vi "1.vi"() -> ()   [LabVIEW 2020]
uses:
  <vilib>/Native 3D Graph/xcontrol/3DPC_SurfacePlot.xctl
  <vilib>/imath/engines/lvmath2/RunTimeEngine/NodeEndStatement/NIMS_NodeEndStatement_Output.vi
  <instcachedir>/0/NIMS_NodeEndStatement_Output_53EC0D466D134D7ABD903AC30B43404B.lvgen/NIMS_NodeEndStatement_Output_53EC0D466D134D7ABD903AC30B43404B_005.vi
  <vilib>/imath/engines/lvmath2/RunTimeEngine/ErrorHandling/NIMS_Finalize Error.vi
  <instcachedir>/0/NIMS_NodeEndStatement_Output_53EC0D466D134D7ABD903AC30B43404B.lvgen/NIMS_NodeEndStatement_Output_53EC0D466D134D7ABD903AC30B43404B_002.vi
panel:
  out "3D Graph 3":refnum<class "Base Datatype.lvclass">[](xcontrol)
  in  "Cutter Height":dbl=10.0
  in  "Cutter Diameter":dbl=20.0
  in  "Thickness":dbl=3.0
  in  "Cylinder Height":dbl=50.0
  in  "Diameter":dbl=60.0
  in  "Number of waves":dbl=4.0
  in  "Amplitude":dbl=6.0
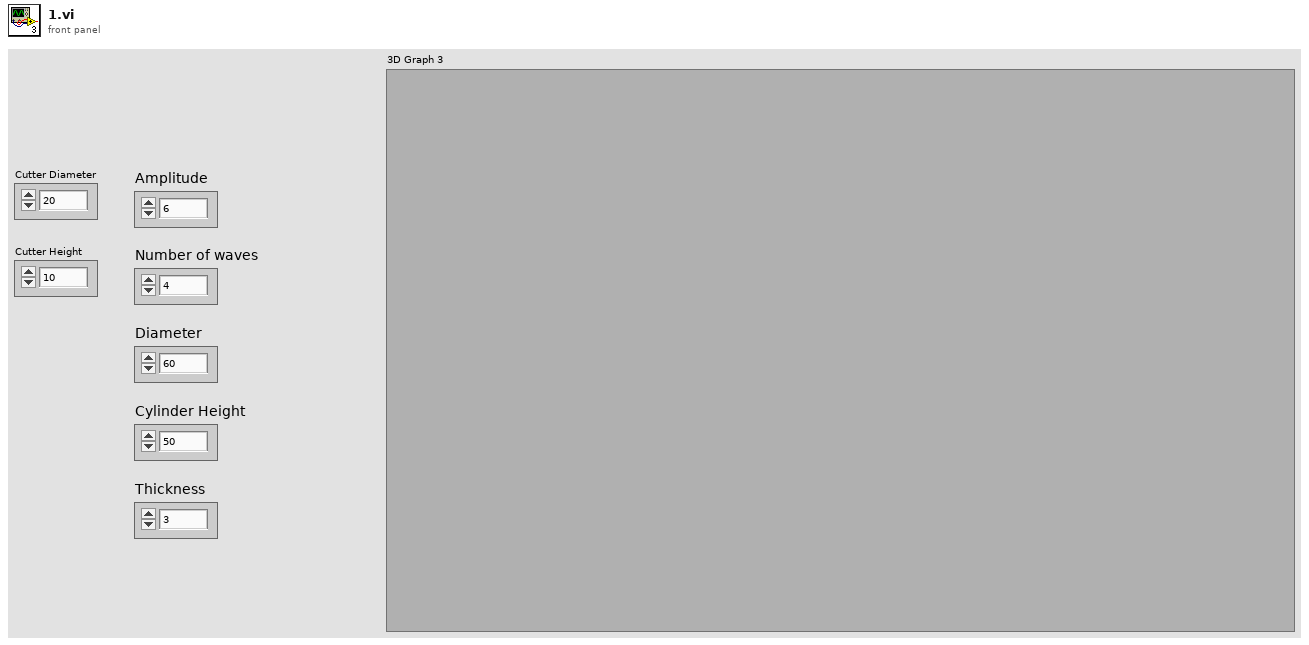
[diagram p1: front panel]
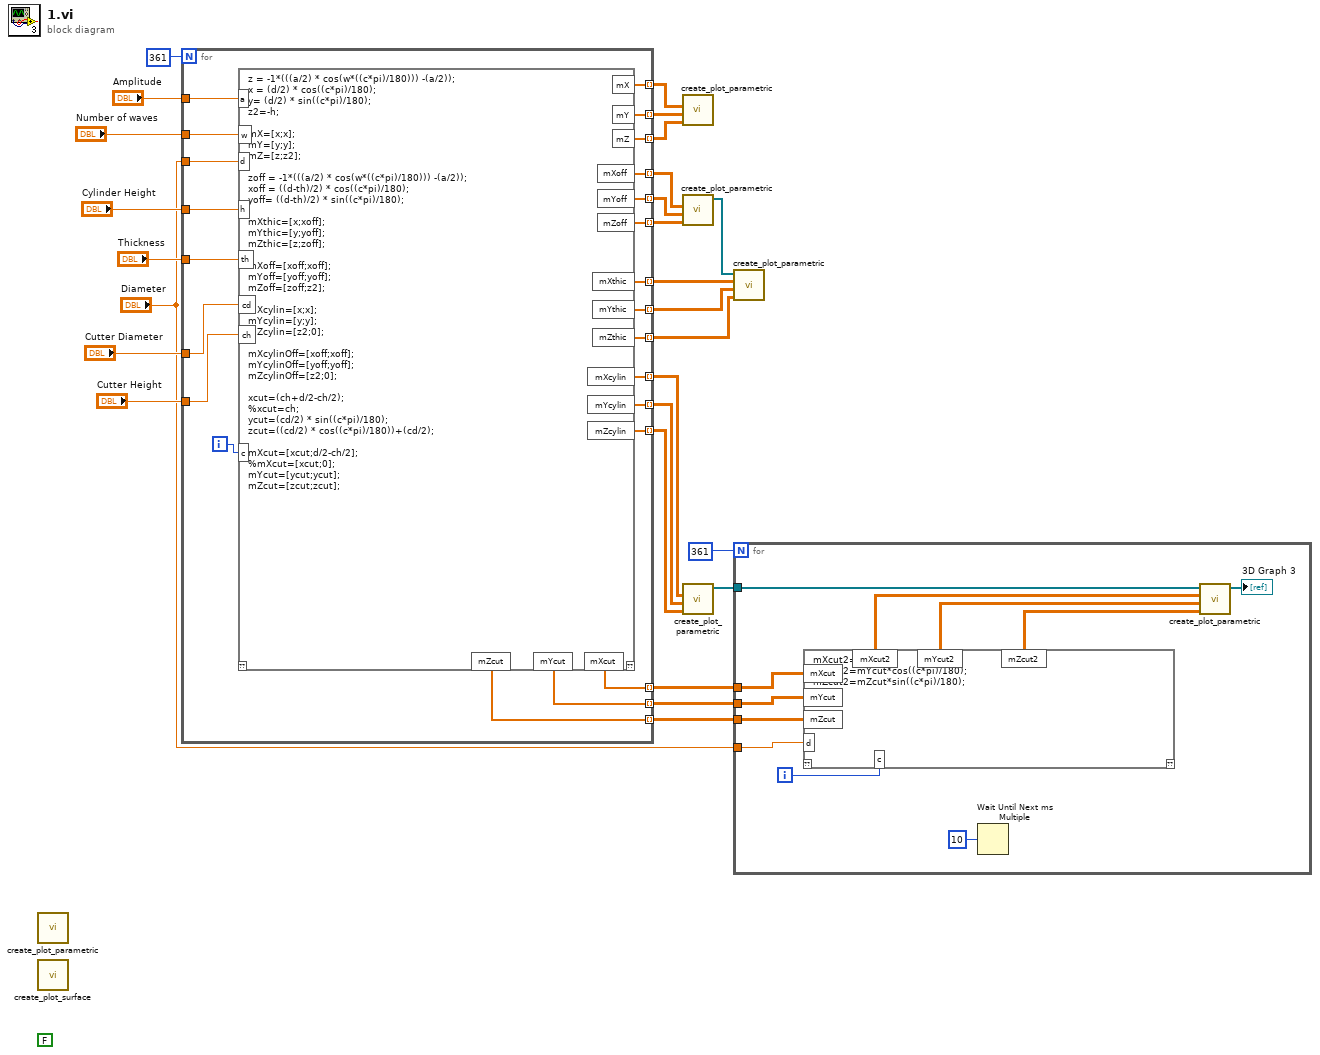
[diagram p0: block diagram]
diagram:
  (unwired) FALSE ("Axes:Grid Visible")
  n1 = call <vilib>:"create_plot_parametric.vi"() -> ()  [unwired: 5 in, 7 out]
  n2 = call <vilib>:"create_plot_surface.vi"() -> ()  [unwired: 5 in, 7 out]
  n3 = for {
    N: 361 -> [_]
    tunnel: "Amplitude" -> [w49]
    tunnel: "Number of waves" -> [w48]
    tunnel: "Diameter" -> [w47]
    tunnel: [w46] -> w20 mode=indexing
    tunnel: [w45] -> w21 mode=indexing
    tunnel: [w44] -> w19 mode=indexing
    tunnel: "Cylinder Height" -> [w42]
    tunnel: [w41] -> w23 mode=indexing
    tunnel: [w40] -> w22 mode=indexing
    tunnel: [w39] -> w13 mode=indexing
    tunnel: [w38] -> w17 mode=indexing
    tunnel: [w37] -> w16 mode=indexing
    tunnel: [w36] -> w15 mode=indexing
    tunnel: "Thickness" -> [w35]
    tunnel: [w34] -> w12 mode=indexing
    tunnel: [w33] -> w11 mode=indexing
    tunnel: [w32] -> w7 mode=indexing
    tunnel: "Cutter Diameter" -> [w31]
    tunnel: "Cutter Height" -> [w30]
    tunnel: [w29] -> w6 mode=indexing
    tunnel: [w28] -> w5 mode=indexing
    tunnel: [w27] -> w4 mode=indexing
    i -> [w43]
    n4 = mathscript code="z = -1*(((a/2) * cos(w*((c*pi)/180))) -(a/2));\nx = (d/2) * cos((c*pi)/180);\ny= (d/2) * sin((c*pi)/180);\nz2=-h;\n\nmX=[x;x];\nmY=[y;y];\nmZ=[z;z2];\n\nzoff = -1*(((a/2) * cos(w*((c*pi)/180))) -(a/2));\nxoff = ((d-th)/2) * cos((c*pi)/180);\nyoff= ((d-th)/2) * sin((c*pi)/180);\n\nmXthic=[x;xoff];\nmYthic=[y;yoff];\nmZthic=[z;zoff];\n\nmXoff=[xoff;xoff];\nmYoff=[yoff;yoff];\nmZoff=[zoff;z2];\n\nmXcylin=[x;x];\nmYcylin=[y;y];\nmZcylin=[z2;0];\n\nmXcylinOff=[xoff;xoff];\nmYcylinOff=[yoff;yoff];\nmZcylinOff=[z2;0];\n\nxcut=(ch+d/2-ch/2);\n%xcut=ch;\nycut=(cd/2) * sin((c*pi)/180);\nzcut=((cd/2) * cos((c*pi)/180))+(cd/2);\n\nmXcut=[xcut;d/2-ch/2];\n%mXcut=[xcut;0];\nmYcut=[ycut;ycut];\nmZcut=[zcut;zcut];"("a"=w49, "w"=w48, "c"=w43, "d"=w47, "h"=w42, "th"=w35, "cd"=w31, "ch"=w30) -> ("mZoff"=w44:dbl[], "mXoff"=w45:dbl[], "mYoff"=w46:dbl[], "mX"=w41:dbl[], "mY"=w40:dbl[], "mZ"=w39:dbl[], "mXthic"=w38:dbl[], "mYthic"=w37:dbl[], "mZthic"=w36:dbl[], "mXcylin"=w34:dbl[], "mYcylin"=w33:dbl[], "mZcylin"=w32:dbl[], "mXcut"=w29:dbl[], "mYcut"=w28:dbl[], "mZcut"=w27:dbl[])  [unwired: 1 in, 1 out]
  }
  n5 = call <vilib>:"create_plot_parametric.vi"("z matrix"=w13, "y matrix"=w22, "x matrix"=w23) -> ()  [unwired: 2 in, 7 out]
  n6 = call <vilib>:"create_plot_parametric.vi"("z matrix"=w19, "y matrix"=w20, "x matrix"=w21) -> ("plots out"=w10:refnum<class "Base Datatype.lvclass">[])  [unwired: 2 in, 6 out]
  n7 = call <vilib>:"create_plot_parametric.vi"("z matrix"=w7, "y matrix"=w11, "x matrix"=w12) -> ("plots out"=w1:refnum<class "Base Datatype.lvclass">[])  [unwired: 2 in, 6 out]
  n8 = call <vilib>:"create_plot_parametric.vi"("z matrix"=w15, "y matrix"=w16, "x matrix"=w17, "plots in"=w10) -> ()  [unwired: 1 in, 7 out]
  n9 = for {
    N: 361 -> [_]
    tunnel: w6 -> [w384]
    tunnel: w5 -> [w381]
    tunnel: w4 -> [w380]
    tunnel: "Diameter" -> [w376]
    tunnel: w1 -> [w375]
    i -> [w385]
    n10 = mathscript code="mXcut2=mXcut;\nmYcut2=mYcut*cos((c*pi)/180);\nmZcut2=mZcut*sin((c*pi)/180);"("mXcut"=w384, "c"=w385, "mYcut"=w381, "mZcut"=w380, "d"=w376) -> ("mXcut2"=w383:dbl[][], "mYcut2"=w379:dbl[][], "mZcut2"=w378:dbl[][])  [unwired: 1 in, 1 out]
    n11 = Wait Until Next ms Multiple(millisecond multiple=u32 10) -> ()  [unwired: 1 out]
    n12 = call <vilib>:"create_plot_parametric.vi"("z matrix"=w378, "y matrix"=w379, "x matrix"=w383, "plots in"=w375) -> ("plots out"=→"3D Graph 3":refnum<class "Base Datatype.lvclass">[])  [unwired: 1 in, 6 out]
  }
